vi "BuildCrossArray.vi"(0 "Plate \nDiameter (mm)":dbl, 2 "Cross X dimension\n(cross is square)":dbl, 3 "Desired\nSpacing(mm)":dbl, 5 "PathSupreme":T1) -> (6 "PathSupreams":T1[](array[typedef]), 7 "Array 2":dbl[][](array[numeric]))   [LabVIEW 2014]
uses:
  Slicer/LVslicer/Slice/TypeDefs/PathSupreme.ctl
  Slicer/LVslicer/Slice/OverhangParam/PSup2SCAN/Sub/VelocityProfile.ctl
  Slicer/LVslicer/Slice/OverhangParam/PSup2SCAN/Sub/PathCut.ctl
  Slicer/LVslicer/Slice/OverhangParam/PSup2SCAN/Sub/Segment.ctl
panel:
  out "Radius max":dbl
  out "Total # \nof crosses":dbl
  out "Gap":dbl
  out "Spacing Used":dbl format="%#.3g"
  out "# of crosses/fill":dbl
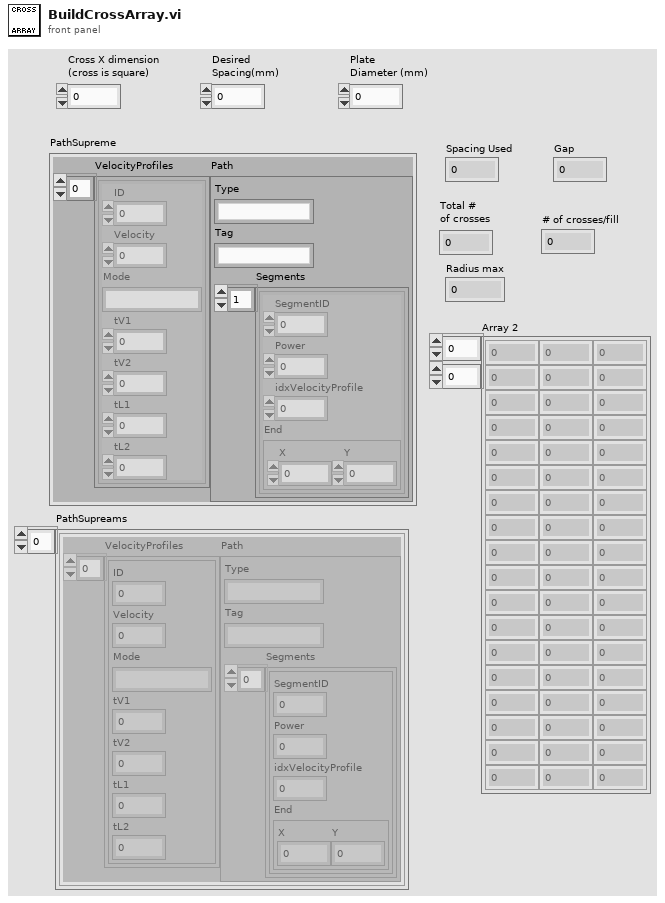
[diagram p1: front panel]
types:
  T1 = typedef "PathSupreme.ctl" = cluster{"VelocityProfiles":T2[], "Path":T3}
  T2 = typedef "VelocityProfile.ctl" = cluster{"ID":u32, "Velocity":dbl, "Mode":string, "tV1":u32, "tV2":u32, "tL1":u32, "tL2":u32}
  T3 = typedef "PathCut.ctl" = cluster{"Type":string, "Tag":string, "Segments":T4[]}
  T4 = typedef "Segment.ctl" = cluster{"SegmentID":u16, "Power":sgl, "idxVelocityProfile":u16, "End":cluster{"X":sgl, "Y":sgl}}
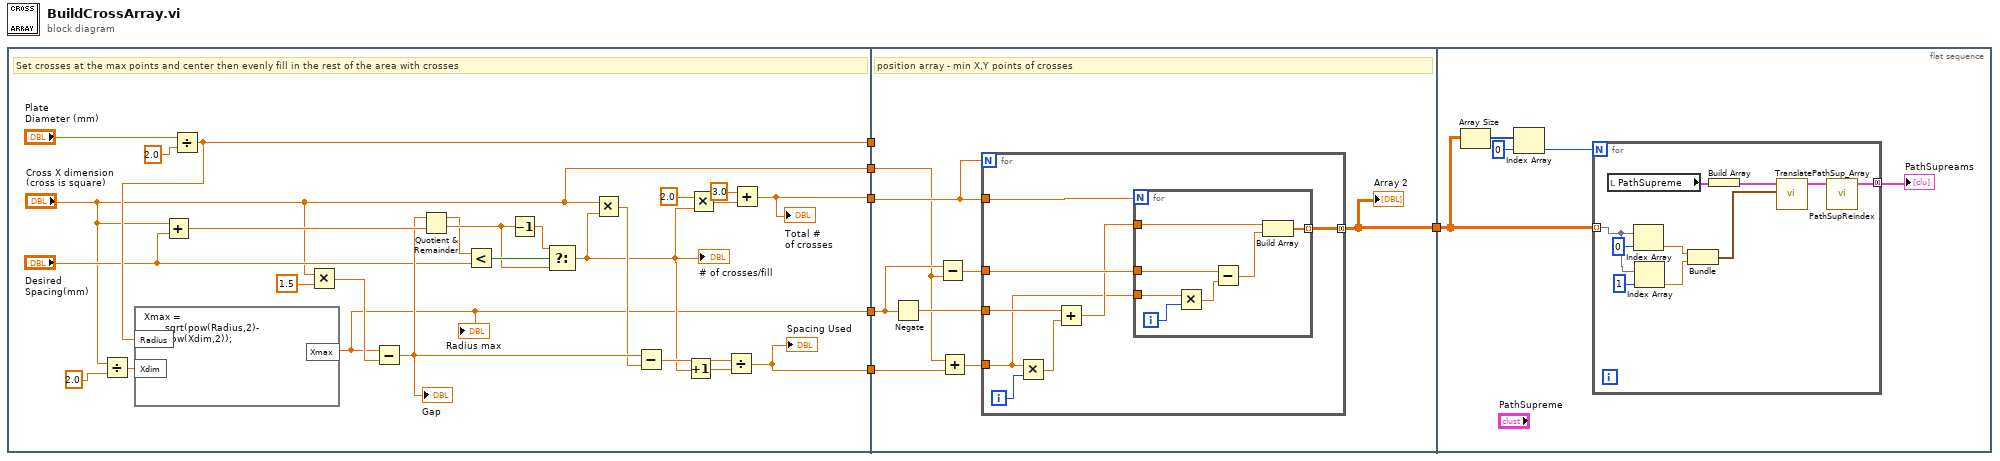
[diagram p0: block diagram]
diagram:
  n1 = flat-sequence {
    tunnel: [w16] -> w6
    tunnel: [w14] -> w5
    tunnel: [w15] -> w4
    tunnel: ["Cross X dimension\n(cross is square)"] -> w3
    tunnel: [w7] -> w1
    tunnel: w6 -> [w35]
    tunnel: w5 -> [_]
    tunnel: w4 -> [w37]
    tunnel: w3 -> [w33]
    tunnel: [w36] -> w2
    tunnel: w1 -> [w34]
    tunnel: w2 -> [w55]
    frame #0 {
      # "Xmax = \"Radius\""
      # "Set crosses at the max points and center then evenly fill in the rest of the area with crosses"
      n2 = Divide(x="Cross X dimension\n(cross is square)", y=2.0) -> (x/y=w8:dbl)
      n3 = Add(x="Cross X dimension\n(cross is square)", y="Desired\nSpacing(mm)") -> (x+y=w31:dbl)
      n4 = Divide(x="Plate \nDiameter (mm)", y=2.0) -> (x/y=w14:dbl)
      n5 = formula code="Xmax = \n       sqrt(pow(Radius,2)-\n       pow(Xdim,2));"("Radius"=w14, "Xdim"=w8) -> ("Xmax"=w15:dbl)
      "Radius max" <- w15
      n6 = Multiply(x="Cross X dimension\n(cross is square)", y=1.5) -> (x*y=w28:dbl)
      n7 = Subtract(x=w15, y=w28) -> (x-y=w30:dbl)
      "Gap" <- w30
      n8 = Quotient & Remainder(x=w30, y=w31) -> (x-y*floor(x/y)=w12:dbl, floor(x/y)=w25:dbl)
      n9 = Less?(x=w12, y="Desired\nSpacing(mm)") -> (x < y?=w27:bool)
      n10 = Decrement(x=w25) -> (x-1=w26:dbl)
      n11 = Select(t=w26, s=w27, f=w25) -> (s? t:f=w19:dbl)
      "# of crosses/fill" <- w19
      n12 = Multiply(x="Cross X dimension\n(cross is square)", y=w19) -> (x*y=w24:dbl)
      n13 = Subtract(x=w30, y=w24) -> (x-y=w23:dbl)
      n14 = Increment(x=w19) -> (x+1=w11:dbl)
      n15 = Multiply(x=2.0, y=w19) -> (x*y=w20:dbl)
      n16 = Divide(x=w23, y=w11) -> (x/y=w7:dbl)
      "Spacing Used" <- w7
      n17 = Add(x=3.0, y=w20) -> (x+y=w16:dbl)
      "Total # \nof crosses" <- w16
    }
    frame #1 {
      # "position array - min X,Y points of crosses"
      n18 = Negate(x=w37) -> (-x=w39:dbl)
      n19 = Subtract(x=w37, y=w33) -> (x-y=w38:dbl)
      n20 = Add(x=w33, y=w34) -> (x+y=w32:dbl)
      n21 = for {
        N: w35 -> [_]
        tunnel: w39 -> [w46]
        tunnel: w35 -> [w45]
        tunnel: w38 -> [w44]
        tunnel: [w42] -> w36 mode=concatenating
        tunnel: w32 -> [w40]
        i -> [w47]
        n22 = Multiply(x=w40, y=w47) -> (x*y=w41:dbl)
        n23 = Add(x=w46, y=w41) -> (x+y=w43:dbl)
        n24 = for {
          N: w45 -> [_]
          tunnel: w44 -> [w52]
          tunnel: w43 -> [w51]
          tunnel: [w49] -> w42 mode=indexing
          tunnel: w40 -> [w48]
          i -> [w54]
          n25 = Multiply(x=w48, y=w54) -> (x*y=w53:dbl)
          n26 = Subtract(x=w52, y=w53) -> (x-y=w50:dbl)
          n27 = Build Array(w51, w50) -> (w49:dbl[])
        }
      }
      "Array 2" <- w36
    }
    frame #2 {
      n28 = Array Size(array=w55) -> (size(s)=w59:i32[])
      n29 = Index Array(array=w59, index=0) -> (element=w57:i32)
      n30 = for {
        N: w57 -> [_]
        tunnel: w55 -> [w69] mode=indexing
        tunnel: [w61] -> w56 mode=concatenating
        n31 = local read "PathSupreme"() -> (w63:T1)
        n32 = Index Array(array=w69, index=0) -> (element=w65:dbl)
        n33 = Index Array(array=w69, index=1) -> (element=w66:dbl)
        n34 = Bundle(w65, w66) -> (w64:cluster{dbl, dbl})  [unwired: 1 in]
        n35 = Build Array(w63) -> (w62:T1[])
        n36 = call "TranslatePathSup_Array.vi"("Offset"=w64, "PathSupsIn"=w62) -> ("PathSupsOut"=w60:T1[])  [unwired: 9 in]
        n37 = call "PathSupReindex.vi"("PathSupremes"=w60) -> ("PathSupOut"=w61:T1[])  [unwired: 10 in]
      }
      "PathSupreams" <- w56
    }
  }
